vi "Create and Queue New Plugin Command.vi"(8 "error in (no error)":errorcluster, 9 "Matching Plugin":T1, 10 "New Plugin":T5, 11 "CIFPluginManager in":refnum<class "CIFPluginManager.lvclass">) -> (0 "error out":errorcluster)   [LabVIEW 2021, in "CIFPluginManager.lvclass"]
uses:
  CIFPluginManager.lvclass
  CIFPluginManager.lvclass/CIFPluginManager.ctl
  gRPC/CIF_Manager_server/RPC Messages/cif_channelcore_ChannelPattern.ctl
  gRPC/CIF_Manager_server/CIF_Manager_server.lvlib
  gRPC/CIF_Manager_server/RPC Messages/cif_channelcore_ChannelDirection.ctl
  gRPC/CIF_Manager_server/RPC Messages/cif_channelcore_Channel.ctl
  gRPC/CIF_Manager_server/RPC Messages/cif_channelcore_Channels.ctl
  gRPC/CIF_Manager_server/RPC Messages/cif_plugincore_MonitorI64.ctl
  gRPC/CIF_Manager_server/RPC Messages/cif_plugincore_MonitorU64.ctl
  gRPC/CIF_Manager_server/RPC Messages/cif_plugincore_MonitorDoubles.ctl
  gRPC/CIF_Manager_server/RPC Messages/cif_plugincore_Error.ctl
  gRPC/CIF_Manager_server/RPC Messages/cif_common_TimingStats.ctl
  gRPC/CIF_Manager_server/RPC Messages/cif_plugincore_FifoStatistics.ctl
  gRPC/CIF_Manager_server/RPC Messages/cif_plugincore_TimingStatistics.ctl
  gRPC/CIF_Manager_server/RPC Messages/cif_plugincore_StatusData_PluginState.ctl
  gRPC/CIF_Manager_server/RPC Messages/cif_plugincore_StatusData.ctl
  CIFCore/Common/Typedef/Version.ctl
  CIFCore/Common/CIFCoreCommon.lvlib
  <vilib>/gRPC/LabVIEW gRPC Library/Shared/grpcId.ctl
  <vilib>/gRPC/LabVIEW gRPC Library/grpc-lvsupport-release.lvlib
  typedef/Plugin Management Data.ctl
  typedef/Loader Type.ctl
  typedef/Plugin Load Info.ctl
  typedef/Plugin Metadata.ctl
  typedef/Discovered Plugin.ctl
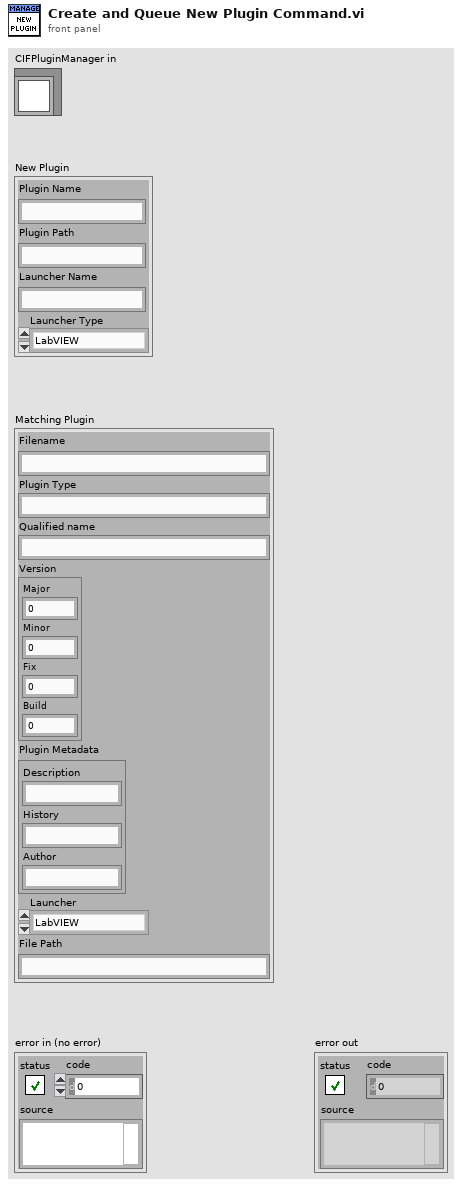
[diagram p1: front panel]
types:
  T1 = typedef "CIFPluginManager.lvclass/Discovered Plugin.ctl" = cluster{"Filename":string, "Plugin Type":string, "Qualified name":string, "Version":T2, "Plugin Metadata":T3, "Launcher":T4, "File Path":string}
  T2 = typedef "CIFCoreCommon.lvlib/Version.ctl" = cluster{"Major":i32, "Minor":i32, "Fix":i32, "Build":i32}
  T3 = typedef "CIFPluginManager.lvclass/Plugin Metadata.ctl" = cluster{"Description":string, "History":string, "Author":string}
  T4 = typedef "CIFPluginManager.lvclass/Loader Type.ctl" = enum16{"LabVIEW"}
  T5 = typedef "CIFPluginManager.lvclass/Plugin Load Info.ctl" = cluster{"Plugin Name":string, "Plugin Path":string, "Launcher Name":string, "Launcher Type":T4}
  T6 = typedef "CIFPluginManager.lvclass/Loader Map.ctl" = map{string, T7}
  T7 = typedef "CIFPluginManager.lvclass/Loaders.ctl" = cluster{"Loader Type":T4, "grpc_port":i32, "pid":u32, "gRPC ID":T8, "Load Timestamp":i64, "Unloading":bool, "Ready for removal":bool, "Unload Timestamp":i64}
  T8 = typedef "grpc-lvsupport-release.lvlib/grpcId.ctl" = u64
  T9 = typedef "CIFPluginManager.lvclass/Plugin Management Data.ctl" = cluster{"vi reference":refnum<vi>, "Launcher":string, "gRPC ID":T8, "Plugin Type":string, "Unique Name":string, "gRPC Port":i32, "Version":T2, "Load Timestamp":i64, "Unload Timestamp":i64, "Unloading":bool, "Ready for removal":bool, "status":T10, "channels":T19}
  T10 = typedef "CIF_Manager_server.lvlib/cif_plugincore_StatusData.ctl" = cluster{"state":T11, "timing_statistics":T12, "fifo_statistics":T14, "error":T15, "monitor_doubles":T16, "monitor_u64s":T17, "monitor_i64s":T18}
  T11 = typedef "CIF_Manager_server.lvlib/cif_plugincore_StatusData_PluginState.ctl" = enum32{"PLUGINSTATE_UNKNOWN", "PLUGINSTATE_CREATING", "PLUGINSTATE_LISTENING", "PLUGINSTATE_RUNNING", "PLUGINSTATE_CLEANINGUP", "PLUGINSTATE_DESTROYING"}
  T12 = typedef "CIF_Manager_server.lvlib/cif_plugincore_TimingStatistics.ctl" = cluster{"period":T13, "wake_error":T13, "execute":T13, "housekeep":T13, "idle":T13, "cleanup":T13, "custom_1":T13, "custom_2":T13}
  T13 = typedef "CIF_Manager_server.lvlib/cif_common_TimingStats.ctl" = cluster{"max":i64, "min":i64, "avg":dbl}
  T14 = typedef "CIF_Manager_server.lvlib/cif_plugincore_FifoStatistics.ctl" = cluster{"from_t0":T13, "from_previous_plugin":T13, "output_error":T13}
  T15 = typedef "CIF_Manager_server.lvlib/cif_plugincore_Error.ctl" = cluster{"status":bool, "code":i32}
  T16 = typedef "CIF_Manager_server.lvlib/cif_plugincore_MonitorDoubles.ctl" = cluster{"double_1":dbl, "double_2":dbl, "double_3":dbl, "double_4":dbl}
  T17 = typedef "CIF_Manager_server.lvlib/cif_plugincore_MonitorU64.ctl" = cluster{"u64_1":u64, "u64_2":u64, "u64_3":u64, "u64_4":u64}
  T18 = typedef "CIF_Manager_server.lvlib/cif_plugincore_MonitorI64.ctl" = cluster{"i64_1":i64, "i64_2":i64, "i64_3":i64, "i64_4":i64}
  T19 = typedef "CIF_Manager_server.lvlib/cif_channelcore_Channels.ctl" = cluster{"channels":T20[]}
  T20 = typedef "CIF_Manager_server.lvlib/cif_channelcore_Channel.ctl" = cluster{"name":string, "direction":T21, "type":string, "custom_config":u8[], "connected":bool, "connected_name":string, "forced":bool, "channel_pattern":T22}
  T21 = typedef "CIF_Manager_server.lvlib/cif_channelcore_ChannelDirection.ctl" = enum32{"CHANNELDIRECTION_UNKNOWN", "CHANNELDIRECTION_PUBLISHER", "CHANNELDIRECTION_SUBSCRIBER"}
  T22 = typedef "CIF_Manager_server.lvlib/cif_channelcore_ChannelPattern.ctl" = enum32{"CHANNELPATTERN_UNKNOWN", "CHANNELPATTERN_TAG", "CHANNELPATTERN_FIFO", "CHANNELPATTERN_MULTIFIFO", "CHANNELPATTERN_BACKPRESSUREFIFO"}
  T23 = typedef "CIFPluginManager.lvclass/Plugin Management Data Map.ctl" = map{string, T9}
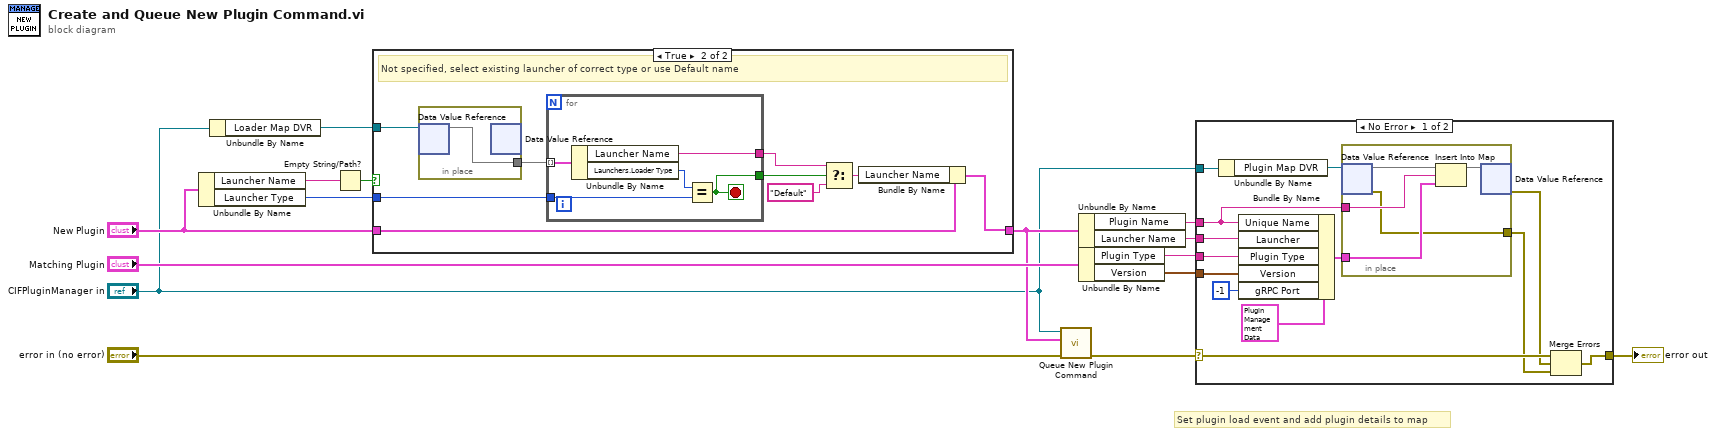
[diagram p0: block diagram]
diagram:
  # "Set plugin load event and add plugin details to map"
  n1 = Unbundle By Name("New Plugin") -> ("Launcher Name"=w3:string, "Launcher Type"=w2:T4)
  n2 = Unbundle By Name("CIFPluginManager in") -> ("Loader Map DVR"=w7:refnum<data-value>)
  n3 = Empty String/Path?(string/path=w3) -> (empty?=w6:bool)
  n4 = case shown="True" w6 {
    tunnel: w7 -> [_ w25]
    tunnel: "New Plugin" -> [w16 w20]
    tunnel: [w16 w18] -> w4
    tunnel: w2 -> [_ w23]
    frame False {
      # "Launcher specified"
    }
    frame True {
      # "Not specified, select existing launcher of correct type or use Default name"
      n5 = in-place {
        in-place-border: [w31] -> w24
        n6 = in-place-dvr #1(w25) -> (w31:T6)  [unwired: 1 out]
        n7 = in-place-dvr #1() -> ()  [unwired: 1 in, 2 out]
      }
      n8 = for {
        tunnel: w24 -> [w30] mode=indexing
        tunnel: w23 -> [w28]
        tunnel: [w27] -> w22
        tunnel: [w26] -> w21
        stop <- w27 stop-if-true
        n9 = Unbundle By Name(w30) -> ("Launcher Name"=w26:string, "Launchers.Loader Type"=w29:T4)
        n10 = Equal?(x=w29, y=w28) -> (x = y?=w27:bool)
      }
      n11 = Select(t=w21, s=w22, f="Default") -> (s? t:f=w19:string)
      n12 = Bundle By Name(cluster=w20, "Launcher Name"=w19) -> (w18:T5)
    }
  }
  n13 = call "Queue New Plugin Command.vi"("error in (no error)"="error in (no error)", "New Plugin"=w4, "CIFPluginManager in"="CIFPluginManager in") -> ("error out"=w14:errorcluster)  [unwired: 8 in]
  n14 = Unbundle By Name(w4) -> ("Plugin Name"=w8:string, "Launcher Name"=w13:string)
  n15 = Unbundle By Name("Matching Plugin") -> ("Plugin Type"=w11:string, "Version"=w10:T2)
  n16 = case shown="No Error" w14 {
    selector: w14 -> [w37 w50]
    tunnel: w13 -> [w33 _]
    tunnel: "CIFPluginManager in" -> [w39 _]
    tunnel: [w34 w50] -> w9
    tunnel: w11 -> [w43 _]
    tunnel: w10 -> [w41 _]
    tunnel: w8 -> [w32 _]
    frame No Error {
      n17 = Unbundle By Name(w39) -> ("Plugin Map DVR"=w38:refnum<data-value>)
      n18 = Bundle By Name(cluster=T9 {"vi reference"=refnum, "Launcher"="", "gRPC ID"=0, "Plugin Type"="", "Unique Name"="", "gRPC Port"=0, "Version"={"Major"=0, "Minor"=0, "Fix"=0, "Build"=0}, "Load Timestamp"=0, "Unload Timestamp"=0, "Unloading"=FALSE, "Ready for removal"=FALSE, "status"={"state"=enum."PLUGINSTATE_UNKNOWN", "timing_statistics"={"period"={"max"=0, "min"=0, "avg"=0.0}, "wake_error"={"max"=0, "min"=0, "avg"=0.0}, "execute"={"max"=0, "min"=0, "avg"=0.0}, "housekeep"={"max"=0, "min"=0, "avg"=0.0}, "idle"={"max"=0, "min"=0, "avg"=0.0}, "cleanup"={"max"=0, "min"=0, "avg"=0.0}, "custom_1"={"max"=0, "min"=0, "avg"=0.0}, "custom_2"={"max"=0, "min"=0, "avg"=0.0}}, "fifo_statistics"={"from_t0"={"max"=0, "min"=0, "avg"=0.0}, "from_previous_plugin"={"max"=0, "min"=0, "avg"=0.0}, "output_error"={"max"=0, "min"=0, "avg"=0.0}}, "error"={"status"=FALSE, "code"=0}, "monitor_doubles"={"double_1"=0.0, "double_2"=0.0, "double_3"=0.0, "double_4"=0.0}, "monitor_u64s"={"u64_1"=0, "u64_2"=0, "u64_3"=0, "u64_4"=0}, "monitor_i64s"={"i64_1"=0, "i64_2"=0, "i64_3"=0, "i64_4"=0}}, "channels"={"channels"=[]}} ("Plugin Management Data"), "Unique Name"=w32, "Launcher"=w33, "Plugin Type"=w43, "Version"=w41, "gRPC Port"=-1) -> (w42:T9)
      n19 = in-place {
        in-place-border: w32 -> [w49]
        in-place-border: w42 -> [w48]
        in-place-border: [w45] -> w36
        n20 = in-place-dvr #2(w38) -> (w47:T23, w45:errorcluster)
        n21 = Insert Into Map(map in=w47, key=w49, value=w48) -> (map out=w46:T23)  [unwired: 2 out]
        n22 = in-place-dvr #2(w46) -> (w35:errorcluster)  [unwired: 1 out]
      }
      n23 = Merge Errors(w37, w35, w36) -> (w34:errorcluster)
    }
    frame Error {
    }
  }
  "error out" <- w9
